vi "2039_hw INAVOpenSensors.vi"(2 "External Accel Analog Channel":T6={"X-Axis"=enum."AI 0", "Y-Axis"=enum."Invalid", "Z-Axis"=enum."Invalid"}, 3 "Use External Accel":bool, 4 "Gyroscope Analog Channel":T11) -> (0 "INAV Sensor Cluster":T10 {"GyroDevRef"."Sample Rate" min=0.25 max=100.0 step=0.25; "AccelerometerDevRef"."Device Address" format="%.0x"; "AccelerometerDevRef"."Accel Range" items=["+/- 2 g", "+/- 4 g", "+/- 8 g", "+/- 16 g"]}, 1 "INAV Not OK":bool)   [LabVIEW 2016, in "2039lib.lvlib"]
uses:
  2039lib.lvlib
  <vilib>/Rock Robotics/SystemInterfaces/AI/FPGA_AIGyroChannel.ctl
  <vilib>/Rock Robotics/WPI/Accelerometer/WPI_AccelerometerAnalogChannels.ctl
  <vilib>/Rock Robotics/SystemInterfaces/AI/FPGA_AIChannel.ctl
  <vilib>/Rock Robotics/WPI/Gyro/WPI_GyroDevRef.ctl
  <vilib>/Rock Robotics/SystemInterfaces/spilib/spi_bus.ctl
  <vilib>/Rock Robotics/WPI/Accelerometer/WPI_AccelerometerDevRef.ctl
  <vilib>/Rock Robotics/WPI/Accelerometer/WPI_AccelerometerScaling.ctl
  <vilib>/Rock Robotics/SystemInterfaces/i2clib/i2c_bus.ctl
  <vilib>/Rock Robotics/WPI/Accelerometer/ADXL345 Range.ctl
  <vilib>/Rock Robotics/WPI/Accelerometer/WPI_AccelerometerADXL345 Axes.ctl
  <vilib>/Rock Robotics/WPI/Gyro/WPI_GyroAnalogOpen.vi
  <vilib>/Rock Robotics/WPI/Accelerometer/InternalAccelerometer/WPI_AccelerometerInternalOpen.vi
  <vilib>/Rock Robotics/WPI/Accelerometer/WPI_AccelerometerAnalogOpen.vi
panel:
  # "Analog"
  # "XRS"
  # "ADXL"
  # "Analog"
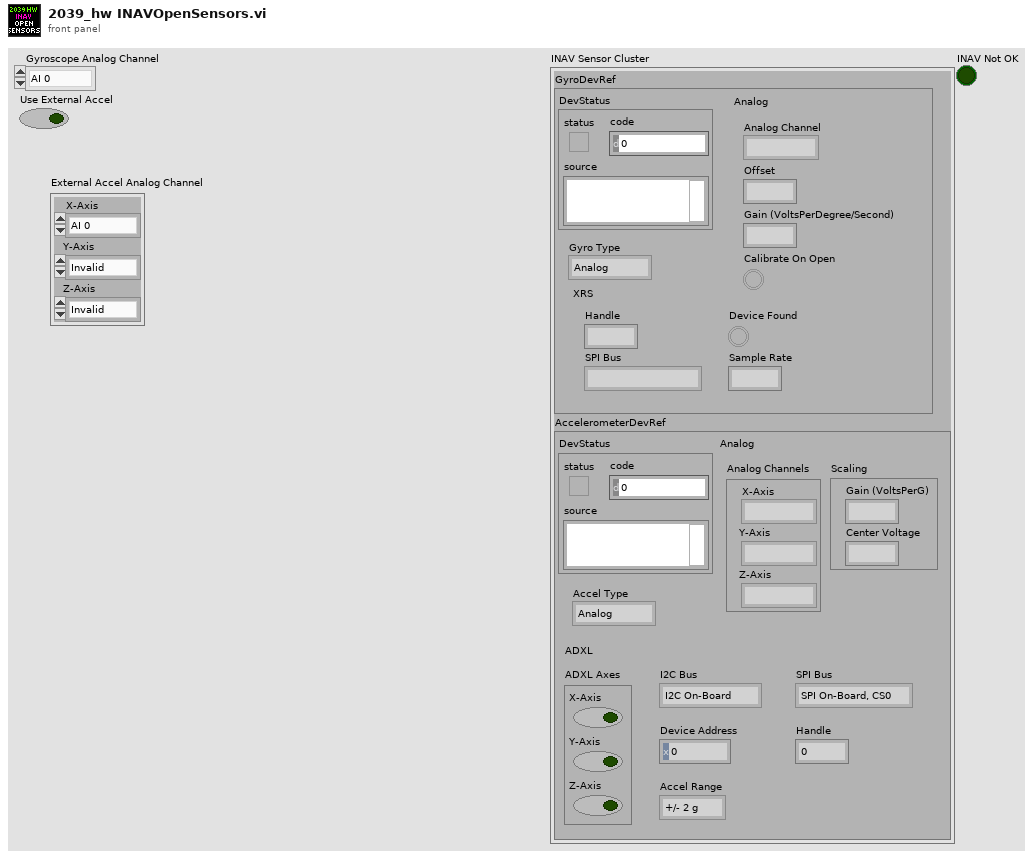
[diagram p1: front panel]
types:
  T1 = typedef "WPI_GyroDevRef.ctl" = cluster{"DevStatus":errorcluster, "Analog Channel":T2, "Offset":dbl, "Gain (VoltsPerDegree/Second)":dbl, "Gyro Type":enum16{"Analog", "XRS450"}, "Handle":i32, "SPI Bus":T3, "Device Found":bool, "Sample Rate":dbl, "Calibrate On Open":bool}
  T2 = typedef "FPGA_AIChannel.ctl" = enum8{"AI 0", "AI 1", "AI 2", "AI 3", "AI MXP 0", "AI MXP 1", "AI MXP 2", "AI MXP 3", "Invalid"}
  T3 = typedef "spi_bus.ctl" = enum16{"SPI On-Board, CS0", "SPI On-Board, CS1", "SPI On-Board, CS2", "SPI On-Board, CS3", "SPI MXP", "Invalid"}
  T4 = typedef "WPI_AccelerometerDevRef.ctl" = cluster{"DevStatus":errorcluster, "Scaling":T5, "Analog Channels":T6, "I2C Bus":T7, "SPI Bus":T3, "Accel Range":T8, "ADXL Axes":T9, "Handle":i32, "Device Address":u8, "Accel Type":enum16{"Analog", "ADXL345 I2C", "ADXL345 SPI", "Internal", "ADXL362 SPI"}}
  T5 = typedef "WPI_AccelerometerScaling.ctl" = cluster{"Gain (VoltsPerG)":dbl, "Center Voltage":dbl}
  T6 = typedef "WPI_AccelerometerAnalogChannels.ctl" = cluster{"X-Axis":T2, "Y-Axis":T2, "Z-Axis":T2}
  T7 = typedef "i2c_bus.ctl" = enum16{"I2C On-Board", "I2C MXP", "Invalid"}
  T8 = typedef "ADXL345 Range.ctl" = u8
  T9 = typedef "WPI_AccelerometerADXL345 Axes.ctl" = cluster{"X-Axis":bool, "Y-Axis":bool, "Z-Axis":bool}
  T10 = cluster{"GyroDevRef":T1, "AccelerometerDevRef":T4}
  T11 = typedef "FPGA_AIGyroChannel.ctl" = enum8{"AI 0", "AI 1", "Invalid"}
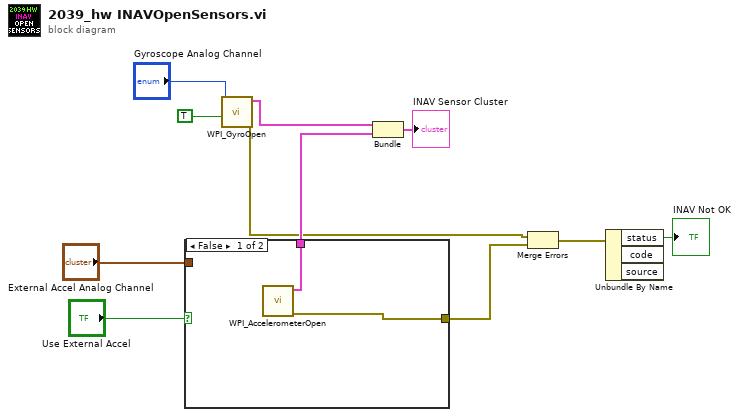
[diagram p0: block diagram]
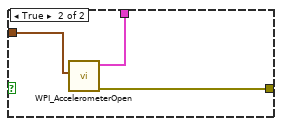
[diagram p2: hidden frame]
diagram:
  n1 = case shown="False" "Use External Accel" {
    tunnel: "External Accel Analog Channel" -> [_ w16]
    tunnel: [w13 w15] -> w6
    tunnel: [w12 w14] -> w3
    frame False {
      n2 = call-poly <vilib>:"WPI_AccelerometerOpen.vi"() -> ("error out"=w12:errorcluster, "AccelerometerDevRef"=w13:T4)  [unwired: 10 in]
    }
    frame True {
      n3 = call-poly <vilib>:"WPI_AccelerometerOpen.vi"("Analog Channels"=w16) -> ("error out"=w14:errorcluster, "AccelerometerDevRef"=w15:T4)  [unwired: 9 in]
    }
  }
  n4 = call-poly <vilib>:"WPI_GyroOpen.vi"("Calibrate On Open"=TRUE, "Analog Channel"="Gyroscope Analog Channel") -> ("error out"=w4:errorcluster, "GyroDevRef"=w9:T1)  [unwired: 7 in, 1 out]
  n5 = Bundle("GyroDevRef"=w9, "AccelerometerDevRef"=w6) -> (→"INAV Sensor Cluster":T10)  [unwired: 1 in]
  n6 = Merge Errors(w4, w3) -> (w2:errorcluster)
  n7 = Unbundle By Name(w2) -> ("status"=→"INAV Not OK":bool)  [unwired: 2 out]
